vi "Generate Value.vi"(8 "error in (no error)":errorcluster, 10 "base value":i64, 11 "variant":variant) -> (0 "error out":errorcluster, 3 "value":variant)   [LabVIEW 2020, in "Value.lvlib"]
uses:
  Value.lvlib
  3336d5e6-6b46-40cc-8581-c00a96048cf3.vi
  c0315305-4ea9-43e2-99a8-a5923f228944.vi
  e9ef65dd-4b85-465f-aa80-4b18505edb13.vi
  babcc117-bc44-41a1-9c2b-73189d1bbfcb.vi
  c68d18eb-9334-419f-972f-f5b5be29402e.vi
  54e220c7-dbf9-4865-aabc-812fe05ebb8b.vi
  47823474-13c3-4f35-a55b-4dd444e3f7d9.vi
  e6de0aaa-8fd3-4213-bbd6-031fb177ed83.vi
  115dbf5b-fdea-438f-8eda-7315cadb6382.vi
  228aee6f-7479-4422-86e8-739061133d5f.vi
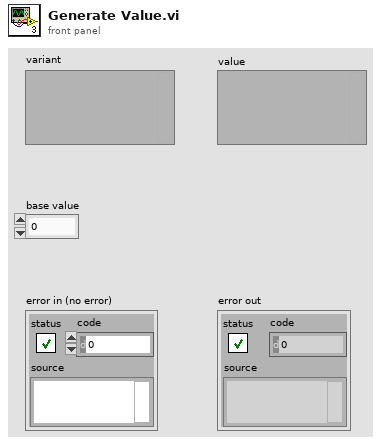
[diagram p1: front panel]
types:
  T1 = typedef "Value.lvlib/Type Code.ctl" = enum8{"Null", "Bool", "BoolA", "Int8", "Int8A", "Int16", "Int16A", "Int32", "Int32A", "Int64", "Int64A", "UInt8", "UInt8A", "UInt16", "UInt16A", "UInt32", "UInt32A", "UInt64", "UInt64A", "Float32", "Float32A", "Float64", "Float64A", "String", "StringA", "Struct", "StructA", "Union", "UnionA", "Any", "AnyA"}
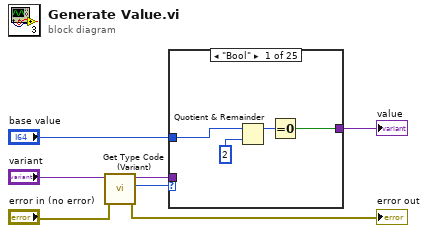
[diagram p0: block diagram]
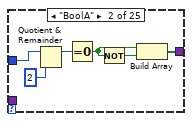
[diagram p2: hidden frame]
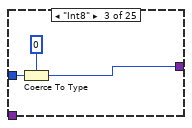
[diagram p3: hidden frame]
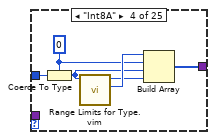
[diagram p4: hidden frame]
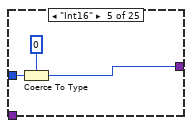
[diagram p5: hidden frame]
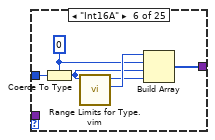
[diagram p6: hidden frame]
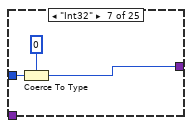
[diagram p7: hidden frame]
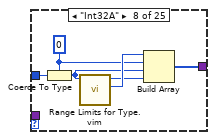
[diagram p8: hidden frame]
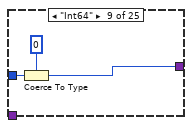
[diagram p9: hidden frame]
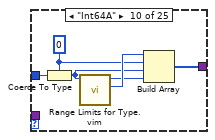
[diagram p10: hidden frame]
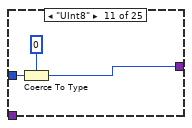
[diagram p11: hidden frame]
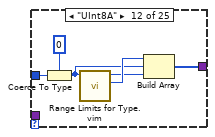
[diagram p12: hidden frame]
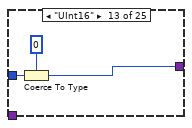
[diagram p13: hidden frame]
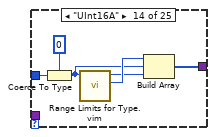
[diagram p14: hidden frame]
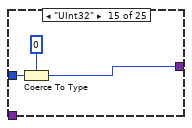
[diagram p15: hidden frame]
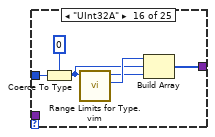
[diagram p16: hidden frame]
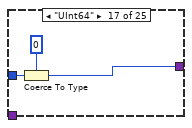
[diagram p17: hidden frame]
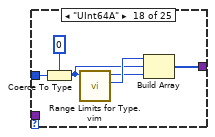
[diagram p18: hidden frame]
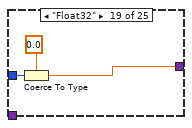
[diagram p19: hidden frame]
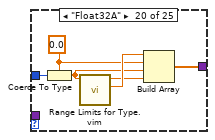
[diagram p20: hidden frame]
diagram:
  n1 = call "Get Type Code (Variant).vi"("error in (no error)"="error in (no error)", "value"="variant") -> ("error out"=→"error out":errorcluster, "type code"=w4:T1, "value dup"=w3:variant)  [unwired: 5 in]
  n2 = case shown="\"Bool\"" w4 {
    tunnel: "base value" -> [w10 w15 w19 w26 w28 w35 w37 w44 w46 w53 w55 w62 w64 w71 w73 w80 w82 w89 w91 w98 w100 w107 w109 w113 _]
    tunnel: [w9 w17 w18 w25 w27 w34 w36 w43 w45 w52 w54 w61 w63 w70 w72 w79 w81 w88 w90 w97 w99 w106 w108 w110 w114] -> w6
    tunnel: w3 -> [_ _ _ _ _ _ _ _ _ _ _ _ _ _ _ _ _ _ _ _ _ _ _ _ w114]
    frame "Bool" {
      n3 = Quotient & Remainder(x=w10, y=i64 2) -> (x-y*floor(x/y)=w8:i64)  [unwired: 1 out]
      n4 = Equal To 0?(x=w8) -> (x = 0?=w9:bool)
    }
    frame "BoolA" {
      n5 = Quotient & Remainder(x=w15, y=i64 2) -> (x-y*floor(x/y)=w14:i64)  [unwired: 1 out]
      n6 = Equal To 0?(x=w14) -> (x = 0?=w12:bool)
      n7 = Not(x=w12) -> (.not. x?=w13:bool)
      n8 = Build Array(w12, w13) -> (w17:bool[])
    }
    frame "Int8" {
      n9 = Coerce To Type(0:w19, 1:i8 0 ("default value")) -> (2:w18:i8)
    }
    frame "Int8A" {
      w22 = i8 0 ("default value")
      n10 = Coerce To Type(0:w26, 1:w22) -> (2:w21:i8)
      n11 = call "Range Limits for Type.vim"("type"=w21) -> ("minimum value for type"=w24:i8, "maximum value for type"=w23:i8)  [unwired: 9 in]
      n12 = Build Array(w24, w22, w21, w23) -> (w25:i8[])
    }
    frame "Int16" {
      n13 = Coerce To Type(0:w28, 1:i16 0 ("default value")) -> (2:w27:i16)
    }
    frame "Int16A" {
      w31 = i16 0 ("default value")
      n14 = Coerce To Type(0:w35, 1:w31) -> (2:w30:i16)
      n15 = call "Range Limits for Type.vim"("type"=w30) -> ("minimum value for type"=w33:i16, "maximum value for type"=w32:i16)  [unwired: 9 in]
      n16 = Build Array(w33, w31, w30, w32) -> (w34:i16[])
    }
    frame "Int32" {
      n17 = Coerce To Type(0:w37, 1:0 ("default value")) -> (2:w36:i32)
    }
    frame "Int32A" {
      w40 = 0 ("default value")
      n18 = Coerce To Type(0:w44, 1:w40) -> (2:w39:i32)
      n19 = call "Range Limits for Type.vim"("type"=w39) -> ("minimum value for type"=w42:i32, "maximum value for type"=w41:i32)  [unwired: 9 in]
      n20 = Build Array(w42, w40, w39, w41) -> (w43:i32[])
    }
    frame "Int64" {
      n21 = Coerce To Type(0:w46, 1:i64 0 ("default value")) -> (2:w45:i64)
    }
    frame "Int64A" {
      w49 = i64 0 ("default value")
      n22 = Coerce To Type(0:w53, 1:w49) -> (2:w48:i64)
      n23 = call "Range Limits for Type.vim"("type"=w48) -> ("minimum value for type"=w51:i64, "maximum value for type"=w50:i64)  [unwired: 9 in]
      n24 = Build Array(w51, w49, w48, w50) -> (w52:i64[])
    }
    frame "UInt8" {
      n25 = Coerce To Type(0:w55, 1:u8 0 ("default value")) -> (2:w54:u8)
    }
    frame "UInt8A" {
      n26 = Coerce To Type(0:w62, 1:u8 0 ("default value")) -> (2:w58:u8)
      n27 = call "Range Limits for Type.vim"("type"=w58) -> ("minimum value for type"=w60:u8, "maximum value for type"=w57:u8)  [unwired: 9 in]
      n28 = Build Array(w60, w58, w57) -> (w61:u8[])
    }
    frame "UInt16" {
      n29 = Coerce To Type(0:w64, 1:u16 0 ("default value")) -> (2:w63:u16)
    }
    frame "UInt16A" {
      n30 = Coerce To Type(0:w71, 1:u16 0 ("default value")) -> (2:w67:u16)
      n31 = call "Range Limits for Type.vim"("type"=w67) -> ("minimum value for type"=w69:u16, "maximum value for type"=w66:u16)  [unwired: 9 in]
      n32 = Build Array(w69, w67, w66) -> (w70:u16[])
    }
    frame "UInt32" {
      n33 = Coerce To Type(0:w73, 1:u32 0 ("default value")) -> (2:w72:u32)
    }
    frame "UInt32A" {
      n34 = Coerce To Type(0:w80, 1:u32 0 ("default value")) -> (2:w76:u32)
      n35 = call "Range Limits for Type.vim"("type"=w76) -> ("minimum value for type"=w78:u32, "maximum value for type"=w75:u32)  [unwired: 9 in]
      n36 = Build Array(w78, w76, w75) -> (w79:u32[])
    }
    frame "UInt64" {
      n37 = Coerce To Type(0:w82, 1:u64 0 ("default value")) -> (2:w81:u64)
    }
    frame "UInt64A" {
      n38 = Coerce To Type(0:w89, 1:u64 0 ("default value")) -> (2:w85:u64)
      n39 = call "Range Limits for Type.vim"("type"=w85) -> ("minimum value for type"=w87:u64, "maximum value for type"=w84:u64)  [unwired: 9 in]
      n40 = Build Array(w87, w85, w84) -> (w88:u64[])
    }
    frame "Float32" {
      n41 = Coerce To Type(0:w91, 1:sgl 0.0 ("default value")) -> (2:w90:sgl)
    }
    frame "Float32A" {
      w94 = sgl 0.0 ("default value")
      n42 = Coerce To Type(0:w98, 1:w94) -> (2:w93:sgl)
      n43 = call "Range Limits for Type.vim"("type"=w93) -> ("minimum value for type"=w96:sgl, "maximum value for type"=w95:sgl)  [unwired: 9 in]
      n44 = Build Array(w96, w94, w93, w95) -> (w97:sgl[])
    }
    frame "Float64" {
      n45 = Coerce To Type(0:w100, 1:0.0 ("default value")) -> (2:w99:dbl)
    }
    frame "Float64A" {
      w103 = 0.0 ("default value")
      n46 = Coerce To Type(0:w107, 1:w103) -> (2:w102:dbl)
      n47 = call "Range Limits for Type.vim"("type"=w102) -> ("minimum value for type"=w105:dbl, "maximum value for type"=w104:dbl)  [unwired: 9 in]
      n48 = Build Array(w105, w103, w102, w104) -> (w106:dbl[])
    }
    frame "String" {
      n49 = Format Value(value (0)=w109) -> (output string=w108:string)  [unwired: 2 in]
    }
    frame "StringA" {
      n50 = Format Value(value (0)=w113) -> (output string=w112:string)  [unwired: 2 in]
      n51 = Build Array(w112, "Hello" ("element")) -> (w110:string[])
    }
    frame Default {
    }
  }
  "value" <- w6
